vi "GetType.vi"(8 "error in (no error)":errorcluster, 11 "StopMovement Msg":refnum<class "StopMovement Msg.lvclass">) -> (0 "error out":errorcluster, 2 "Data Sample":variant, 3 "StopMovement Msg":refnum<class "StopMovement Msg.lvclass">)   [LabVIEW 2015, in "CS++Motor.lvlib" / "StopMovement Msg.lvclass"]
uses:
  StopMovement Msg.lvclass
  StopMovement Msg.lvclass/StopMovement Msg.ctl
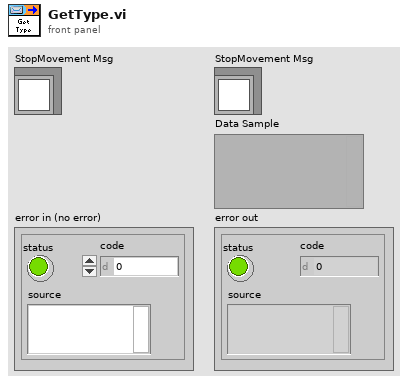
[diagram p1: front panel]
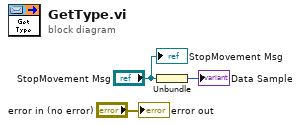
[diagram p0: block diagram]
diagram:
  n1 = Unbundle("StopMovement Msg") -> (→"Data Sample":u8)
  "error out" <- "error in (no error)"
  "StopMovement Msg" <- "StopMovement Msg"
